vi "Configure OVP.vi"(8 "error in (no error)":errorcluster, 9 "Limit (22.0 Volts)":dbl=22.0 format="%.2p", 10 "OVP Enabled (T: On)":bool=TRUE, 11 "VISA resource name":refnum<visa-resource-name>) -> (0 "error out":errorcluster, 3 "VISA resource name out":refnum<visa-resource-name>)   [LabVIEW 2017, in "Agilent E364X Series.lvlib"]
doc: "This VI configures the power supply's over-voltage protection. You specify the over-voltage limit and the behavior of the power supply when the output voltage is greater than or equal to that value."
uses:
  Agilent E364X Series.lvlib
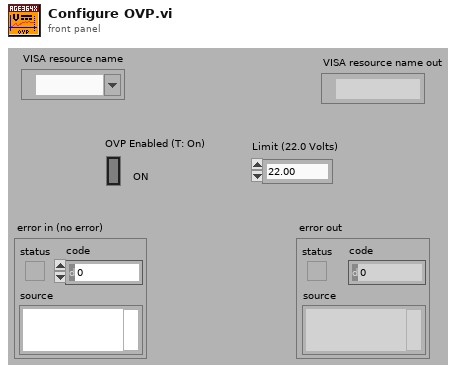
[diagram p1: front panel]
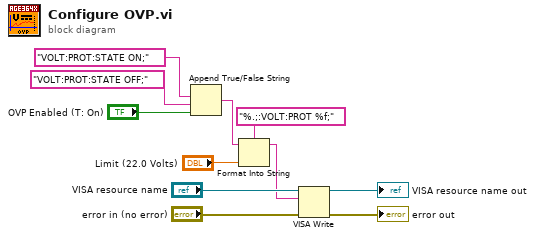
[diagram p0: block diagram]
diagram:
  n1 = Append True/False String(1:"OVP Enabled (T: On)", 2:"VOLT:PROT:STATE OFF;" ("true string"), 3:"VOLT:PROT:STATE ON;" ("true string")) -> (0:w3:string)  [unwired: 1 in]
  n2 = Format Into String(format string="%.;:VOLT:PROT %f;", initial string=w3, "Limit (22.0 Volts)") -> (resulting string=w1:string)  [unwired: 1 in, 1 out]
  n3 = VISA Write(VISA resource name="VISA resource name", write buffer=w1, error in (no error)="error in (no error)") -> (VISA resource name out=→"VISA resource name out":refnum<visa-resource-name>, error out=→"error out":errorcluster)  [unwired: 1 out]
